vi "Patch Folder Gen.vi"(9 "No of Patches":i32, 11 "Experimental Folder":path) -> (0 "Green":path[](array[path]), 2 "Red":path[](array[path]), 3 "Cancelled":bool)   [LabVIEW 2017]
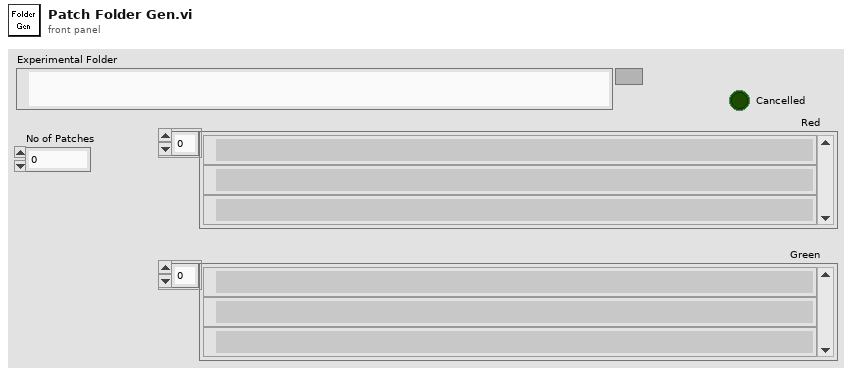
[diagram p1: front panel]
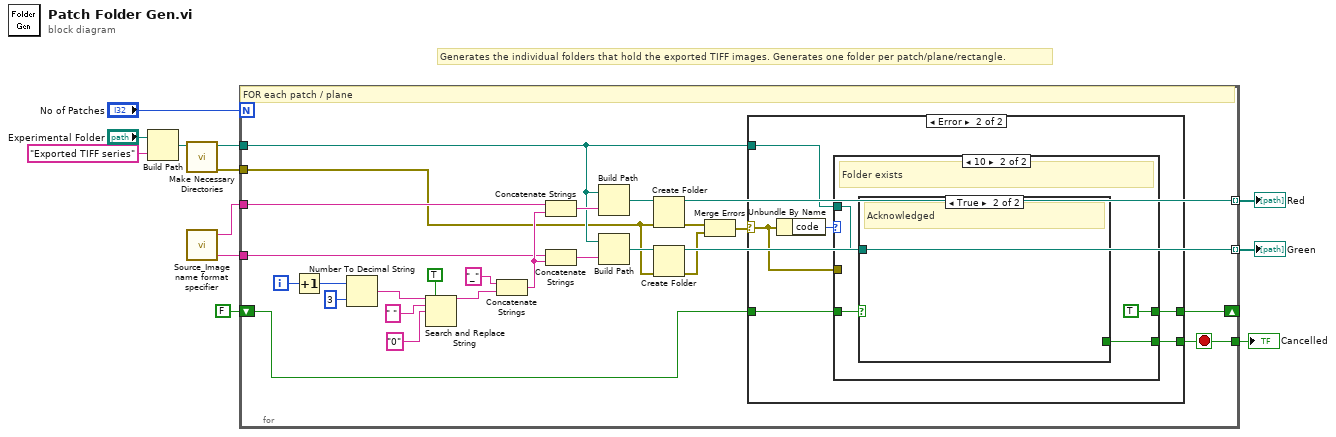
[diagram p0: block diagram]
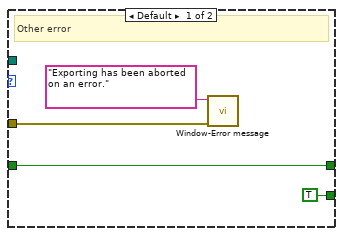
[diagram p3: hidden frame]
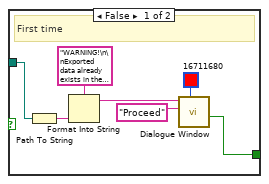
[diagram p4: hidden frame]
diagram:
  # "Generates the individual folders that hold the exported TIFF images. Generates one folder per patch/plane/rectangle."
  n1 = Build Path(base path="Experimental Folder", name or relative path="Exported TIFF series") -> (appended path=w3:path)
  n2 = call <userlib>:"Make Necessary Directories.vi"("Path"=w3) -> ("error out"=w1:errorcluster, "Duplicated path"=w2:path)  [unwired: 9 in]
  n3 = call "Source_Image name format specifier.vi"() -> ("Red channel name"=w11:string, "Green channel name"=w10:string)  [unwired: 5 in, 1 out]
  n4 = for {
    N: "No of Patches" -> [_]
    tunnel: w2 -> [w15]
    tunnel: w11 -> [w28]
    tunnel: w10 -> [w29]
    tunnel: [w22] -> w8 mode=indexing
    tunnel: [w21] -> w9 mode=indexing
    shift-right: [w17] -> _
    shift-left: FALSE -> [w16]
    tunnel: [w14] -> w6
    tunnel: w1 -> [w13]
    i -> [w38]
    stop <- w14 stop-if-true
    # "FOR each patch / plane"
    n5 = Increment(x=w38) -> (x+1=w27:i32)
    n6 = Number To Decimal String(number=w27, width (-)=i16 3) -> (decimal integer string=w36:string)
    n7 = Search and Replace String(replace all?=TRUE ("replace all? (F)"), input string=w36, search string=" ", replace string="0" ("replace string (\"\")")) -> (result string=w32:string)  [unwired: 4 in, 3 out]
    n8 = Concatenate Strings("_" ("string"), w32) -> (w30:string)
    n9 = Concatenate Strings(w28, w30) -> (w26:string)
    n10 = Concatenate Strings(w29, w30) -> (w25:string)
    n11 = Build Path(base path=w15, name or relative path=w26) -> (appended path=w24:path)
    n12 = Build Path(base path=w15, name or relative path=w25) -> (appended path=w23:path)
    n13 = Create Folder(path (use dialog)=w24, error in=w13) -> (created path=w22:path, error out=w20:errorcluster)  [unwired: 1 in, 1 out]
    n14 = Create Folder(path (use dialog)=w23, error in=w13) -> (created path=w21:path, error out=w19:errorcluster)  [unwired: 1 in, 1 out]
    n15 = Merge Errors(w20, w19) -> (w18:errorcluster)
    n16 = case shown="Error" w18 {
      selector: w18 -> [_ w40]
      tunnel: [w39 w44] -> w17
      tunnel: w16 -> [w39 w43]
      tunnel: w15 -> [_ w42]
      tunnel: [_ w41] -> w14
      frame No Error {
      }
      frame Error {
        n17 = Unbundle By Name(w40) -> ("code"=w45:i32)
        n18 = case shown="10" w45 {
          tunnel: [w49 TRUE] -> w44
          tunnel: w43 -> [w49 w52]
          tunnel: w42 -> [_ w51]
          tunnel: [TRUE ("Cancelled (Left button pressed)") w50] -> w41
          tunnel: w40 -> [w47 _]
          frame Default {
            # "Other error"
            n19 = call "Window-Error message.vi"("error in (no error)"=w47, "Message"="Exporting has been aborted on an error.") -> ()  [unwired: 9 in, 1 out]
          }
          frame 10 {
            # "Folder exists"
            n20 = case shown="True" w52 {
              tunnel: w51 -> [w58 _]
              tunnel: [w54 _] -> w50
              frame False {
                # "First time"
                n21 = Path To String(path=w58) -> (string=w56:string)
                n22 = Format Into String(format string="WARNING!\n\nExported data already exists in the following folder. If you proceed exported data will be overwritten.\n\n%s\n" ("Message string"), w56) -> (resulting string=w55:string)  [unwired: 2 in, 1 out]
                n23 = call "Dialogue Window.vi"("Colour"=u32 16711680, "Caption-Right button (OK)"="Proceed", "Message string"=w55) -> ("Cancelled (Left button pressed)"=w54:bool)  [unwired: 6 in, 2 out]
              }
              frame True {
                # "Acknowledged"
              }
            }
          }
        }
      }
    }
  }
  "Green" <- w9
  "Red" <- w8
  "Cancelled" <- w6
